vi "Launcher.vi"() -> ()   [LabVIEW 2021]
uses:
  Root Panel/Root Panel Actor/Root Panel Actor.lvclass
  C:/Program Files (x86)/National Instruments/LabVIEW 2021/vi.lib/MGI/Panel Manager/Panel Actor/Panel Actor/Panel Actor.lvclass
  <vilib>/MGI/Panel Manager/Panel/Window Position/Reference Position/Ref Display/Ref Display.lvclass
  C:/Program Files (x86)/National Instruments/LabVIEW 2021/vi.lib/MGI/Panel Manager/Panel/Window Position/Window Position.lvclass
  <vilib>/MGI/Panel Manager/Panel/Window Position/Reference Position/Ref Display/Ref Display.vi
  <vilib>/MGI/Panel Manager/Panel Actor/Panel Actor/Launch Root Panel Window.vi
  <vilib>/MGI/Monitored Actor/Actor Monitor/Actor Monitor/Actor Monitor.lvclass
  Appearance Actor/Layout Classes/Layout/Layout.lvclass
  <vilib>/MGI/Monitored Actor/Monitored Actor.lvlib
  <vilib>/MGI/Panel Manager/Panel Actor/Panel Actor/Panel Actor.lvclass
  <vilib>/MGI/Panel Manager/Panel/Panel.lvlib
  Appearance Actor/Appearance Actor/Appearance Actor.lvclass
  Appearance Actor/Layout Classes/Predifined Layout/Top Window/API/New Top Window Layout.vi
  Appearance Actor/Layout Classes/Predifined Layout/Top Window/Top Window.lvclass
  C:/Users/Thomas/Documents/Projects/TemplateVIEW/Sources/Appearance Actor/Appearance Actor/Appearance Actor.lvclass
  C:/Program Files (x86)/National Instruments/LabVIEW 2021/vi.lib/MGI/Monitored Actor/Monitored Actor/Monitored Actor/Monitored Actor.lvclass
  C:/Program Files (x86)/National Instruments/LabVIEW 2021/vi.lib/ActorFramework/Actor/Actor.lvclass
  C:/Users/Thomas/Documents/Projects/TemplateVIEW/Sources/Application/Root Panel/Root Panel Actor/Root Panel Actor.lvclass
  C:/Program Files (x86)/National Instruments/LabVIEW 2021/vi.lib/MGI/Panel Manager/Panel/Window Position/Reference Position/Reference Position.lvclass
  C:/Program Files (x86)/National Instruments/LabVIEW 2021/vi.lib/MGI/Panel Manager/Panel/Window Position/Reference Position/Ref Display/Ref Display.lvclass
panel:
  in  "Monitored":bool=TRUE
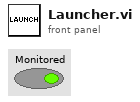
[diagram p1: front panel]
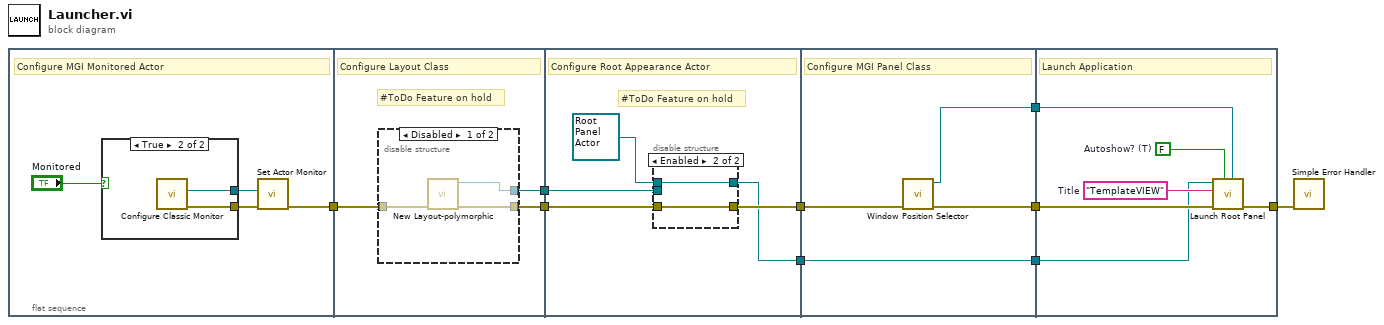
[diagram p0: block diagram]
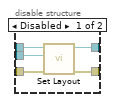
[diagram p4: hidden frame]
diagram:
  n1 = flat-sequence {
    tunnel: [w10] -> w2
    tunnel: [w18] -> w7
    tunnel: [w17] -> w3
    tunnel: w2 -> [w16]
    tunnel: w7 -> [w26]
    tunnel: [w25] -> w9
    tunnel: [w23] -> w4
    tunnel: w3 -> [w24]
    tunnel: w9 -> [w38]
    tunnel: [w37] -> w8
    tunnel: [w36] -> w6
    tunnel: [w35] -> w5
    tunnel: w4 -> [w35]
    tunnel: w8 -> [w42]
    tunnel: w6 -> [w41]
    tunnel: w5 -> [w40]
    tunnel: [w39] -> w1
    frame #0 {
      # "Configure MGI Monitored Actor"
      n2 = case shown="True" "Monitored" {
        tunnel: [_ w15] -> w13
        tunnel: [_ w14] -> w12
        frame False {
        }
        frame True {
          n3 = call <vilib>:"Configure Classic Monitor.vi"() -> ("error out"=w14:errorcluster, "Classic Monitor out"=w15:refnum<class "Actor Monitor.lvclass">)  [unwired: 10 in]
        }
      }
      n4 = call <vilib>:"Set Actor Monitor.vi"("error in (no error)"=w12, "Actor Monitor"=w13) -> ("error out"=w10:errorcluster)  [unwired: 9 in]
    }
    frame #1 {
      # "#ToDo Feature on hold"
      # "Configure Layout Class"
      n5 = disable-structure shown="Disabled" {
        disable-tunnel: w16 -> [w21 w22]
        disable-tunnel: [w20 w22] -> w18
        disable-tunnel: [w19 _] -> w17
        frame Disabled {
          n6 = call-poly "New Layout-polymorphic.vi"("Error In"=w21) -> ("Error Out"=w20:errorcluster, "Top Window Layout"=w19:refnum<class "Layout.lvclass">)  [unwired: 9 in]
        }
        frame Enabled {
        }
      }
    }
    frame #2 {
      # "#ToDo Feature on hold"
      # "Configure Root Appearance Actor"
      n7 = disable-structure shown="Enabled" {
        disable-tunnel: refnum<class "Root Panel Actor.lvclass"> refnum ("Root Panel.lvlib:Root Panel Actor.lvclass") -> [w32 w34]
        disable-tunnel: w26 -> [w31 w33]
        disable-tunnel: [w30 w33] -> w25
        disable-tunnel: w24 -> [w29 _]
        disable-tunnel: [w28 w34] -> w23
        frame Disabled {
          n8 = call "Set Layout.vi"("error in (no error)"=w31, "Layout"=w29, "Appearance Actor in"=w32) -> ("error out"=w30:errorcluster, "Appearance Actor out"=w28:refnum<class "Root Panel Actor.lvclass">)  [unwired: 7 in]
        }
        frame Enabled {
        }
      }
    }
    frame #3 {
      # "Configure MGI Panel Class"
      n9 = call-poly <vilib>:"Window Position Selector.vi"("Error In"=w38) -> ("Error Out"=w37:errorcluster, "Ref Display out"=w36:refnum<class "Ref Display.lvclass">)  [unwired: 9 in]
    }
    frame #4 {
      w44 = FALSE  # Autoshow? (T)
      w43 = "TemplateVIEW"  # Title
      # "Launch Application"
      n10 = call-poly <vilib>:"Launch Root Panel.vi"("Window Position (Maximize First Call)"=w41, "Autoshow? (T)"=w44, "Error In"=w42, "Title"=w43, "Panel Actor in"=w40) -> ("Error Out"=w39:errorcluster)  [unwired: 5 in, 1 out]
    }
  }
  n11 = call <vilib>:"Simple Error Handler.vi"("error in (no error)"=w1) -> ()  [unwired: 4 in, 5 out]
